vi "Acourse_Read Group.vi"(8 "error in (no error)":errorcluster, 11 "Cluster in":T1) -> (0 "error out":errorcluster, 3 "Cluster out":T1)   [LabVIEW 2020]
uses:
  DAQLoop_Typedef.ctl
  controls/DAQ FGV.ctl
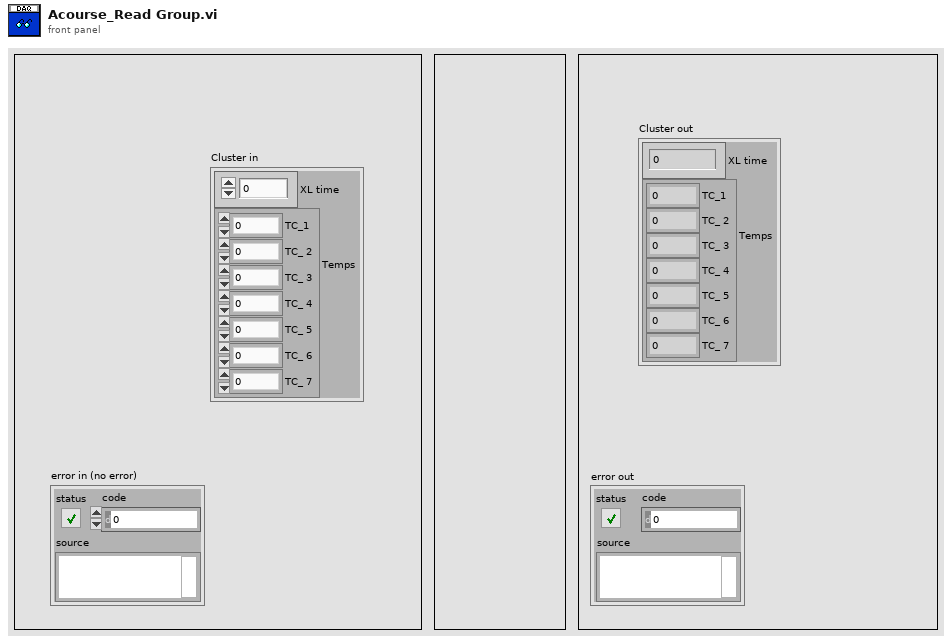
[diagram p1: front panel]
types:
  T1 = typedef "DAQLoop_Typedef.ctl" = cluster{"XL time":dbl, "Temps":cluster{"TC_1":dbl, "TC_ 2":dbl, "TC_ 3":dbl, "TC_ 4":dbl, "TC_ 5":dbl, "TC_ 6":dbl, "TC_ 7":dbl}}
  T2 = typedef "DAQ FGV.ctl" = enum16{"Read", "Pass"}
  T3 = cluster{"TC_1":dbl, "TC_ 2":dbl, "TC_ 3":dbl, "TC_ 4":dbl, "TC_ 5":dbl, "TC_ 6":dbl, "TC_ 7":dbl}
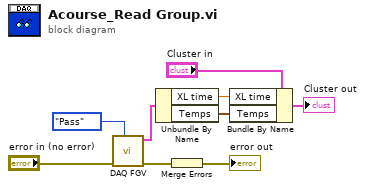
[diagram p0: block diagram]
diagram:
  n1 = call "DAQ FGV.vi"("Enum"=DAQ_FGV."Pass", "error in (no error)"="error in (no error)") -> ("error out"=w6:errorcluster, "Cluster Out"=w3:T1)  [unwired: 8 in]
  n2 = Unbundle By Name(w3) -> ("XL time"=w2:dbl, "Temps"=w1:T3)
  n3 = Merge Errors(w6) -> (→"error out":errorcluster)
  n4 = Bundle By Name(cluster="Cluster in", "XL time"=w2, "Temps"=w1) -> (→"Cluster out":T1)
